vi "HandleCollector.vi"(8 "error in":errorcluster, 9 "JoystickValue":dbl) -> (0 "error out":errorcluster, 1 "CollectorEnum Input":T1)   [LabVIEW 2013]
doc: "Takes in the joystick numeric values and decides whether to raise or lower the collector. Outputs the Collector State enum for raise or lower."
uses:
  CollectorAction.ctl
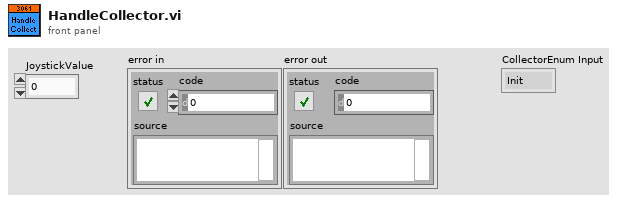
[diagram p1: front panel]
types:
  T1 = typedef "CollectorAction.ctl" = enum16{"Init", "Raise", "Lower", "Stop", "GetStatus"}
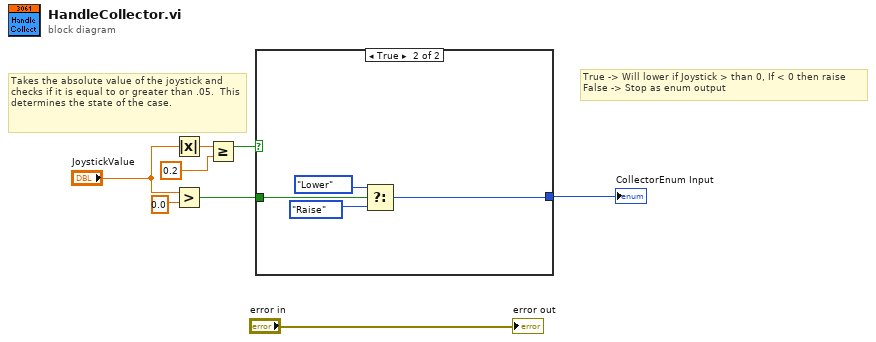
[diagram p0: block diagram]
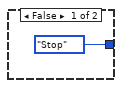
[diagram p2: hidden frame]
diagram:
  # "True -> Will lower if Joystick > than 0, If < 0 then raise\nFalse -> Stop as enum output"
  # "Takes the absolute value of the joystick and checks if it is equal to or greater than .05.  This determines the state of the case."
  n1 = Absolute Value(x="JoystickValue") -> (abs(x)=w7:dbl)
  n2 = Greater?(x="JoystickValue", y=0.0) -> (0:w5:bool)
  n3 = Greater Or Equal?(x=w7, y=0.2) -> (x >= y?=w2:bool)
  n4 = case shown="True" w2 {
    tunnel: [CollectorAction."Stop" ("Enum") w13] -> w8
    tunnel: w5 -> [_ w12]
    frame False {
    }
    frame True {
      n5 = Select(t=CollectorAction."Lower" ("Enum"), s=w12, f=CollectorAction."Raise" ("Enum")) -> (s? t:f=w13:T1)
    }
  }
  "CollectorEnum Input" <- w8
  "error out" <- "error in"
